vi "Save_Setup_File.vi"(1 "Setup filename":string) -> (0 "Setup String":string)   [LabVIEW 2022 SP3]
uses:
  File/Setup_Filetype.ctl
  Globals/Meas_global.vi
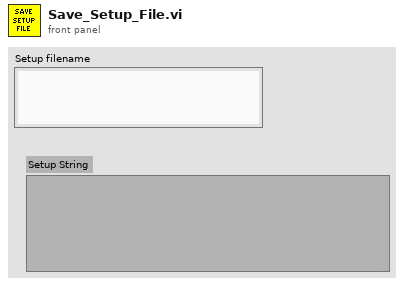
[diagram p1: front panel]
types:
  T1 = typedef "Setup_Filetype.ctl" = enum16{"Measurement Setups", "Calibration Setups", "General", "Results File Plotter Setups", "Speed Calib Tweaks"}
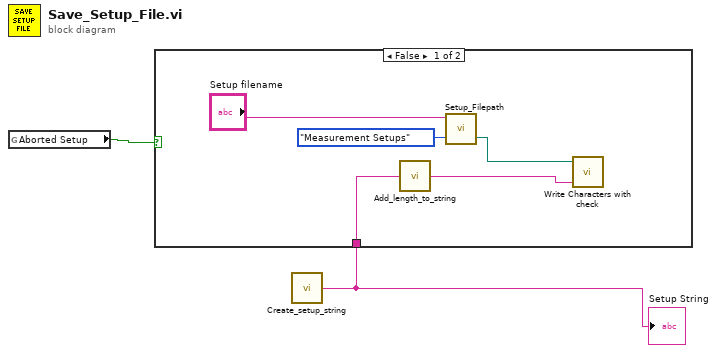
[diagram p0: block diagram]
diagram:
  n1 = global read "Meas_global.vi" "Aborted Setup"() -> (w1:bool)
  n2 = call "Create_setup_string.vi"() -> ("Setup String"=w2:string)  [unwired: 1 out]
  "Setup String" <- w2
  n3 = case shown="False" w1 {
    tunnel: w2 -> [w5 _]
    frame False {
      n4 = call "Add_length_to_string.vi"("String in"=w5) -> ("String out"=w3:string)
      n5 = call "Setup_Filepath.vi"("Setup File Type"=Setup_Filetype."Measurement Setups", "Filename in"="Setup filename") -> ("Filename Out"=w4:path)  [unwired: 1 out]
      n6 = call "Write Characters with check.vi"("String to Write"=w3, "file (use dialog)"=w4) -> ()  [unwired: 2 in, 1 out]
    }
    frame True {
    }
  }
